vi "DTMF_final_rev2.vi"() -> ()   [LabVIEW 2018]
uses:
  <vilib>/Analysis/3filter.llb/Filter Passband Type.ctl
  <vilib>/Analysis/5stat.llb/RMS (DBL).vi
  <vilib>/express/express analysis/Spectral/Block/exnSpectralBlock spectral measurements power poly.vi
  <vilib>/express/express analysis/Spectral/Block/exnSpectralBlock spectral measurements power WFM.vi
  <vilib>/Analysis/3filter.llb/Butterworth Filter (DBL).vi
  <vilib>/express/express analysis/Spectral/XNode/ExpressSpectralMeasurementsBlockNode.xnode
  <vilib>/Analysis/NI_AALPro.lvlib
  <vilib>/Analysis/NI_AALBase.lvlib
panel:
  out "Peaks":cluster{"f0":dbl, "df":dbl, "magnitude":dbl[]}(graph)
  out "Dectected Phone Number!":i32[](array[numeric])
  out "Current Piece of Waveform Graph":dbl[](graph)
  out "appended array 2":dbl[](array[numeric])
  out "Total Signals":dynamicdata(graph) caption="Signals"
  out "max index(es) 2":i32
  out "max index(es)":i32
  out "appended array":dbl[](array[numeric])
  out "rms value":dbl format="%0.2f"
  in  "Emergency Exit":bool
  out "File Directory":path
  # "Tom's Dual Tone Multi Frequency"
  # "<- Total Dialed Phone #"
  # "Represents\ntotal signal ->"
  # "867-5309"
  # "OU SWAG"
  # "<-  Represents two peaks \n      if the phone number \n      is pressed"
  # "Represents how the \nwaveform looks in\nthe graph            ->"
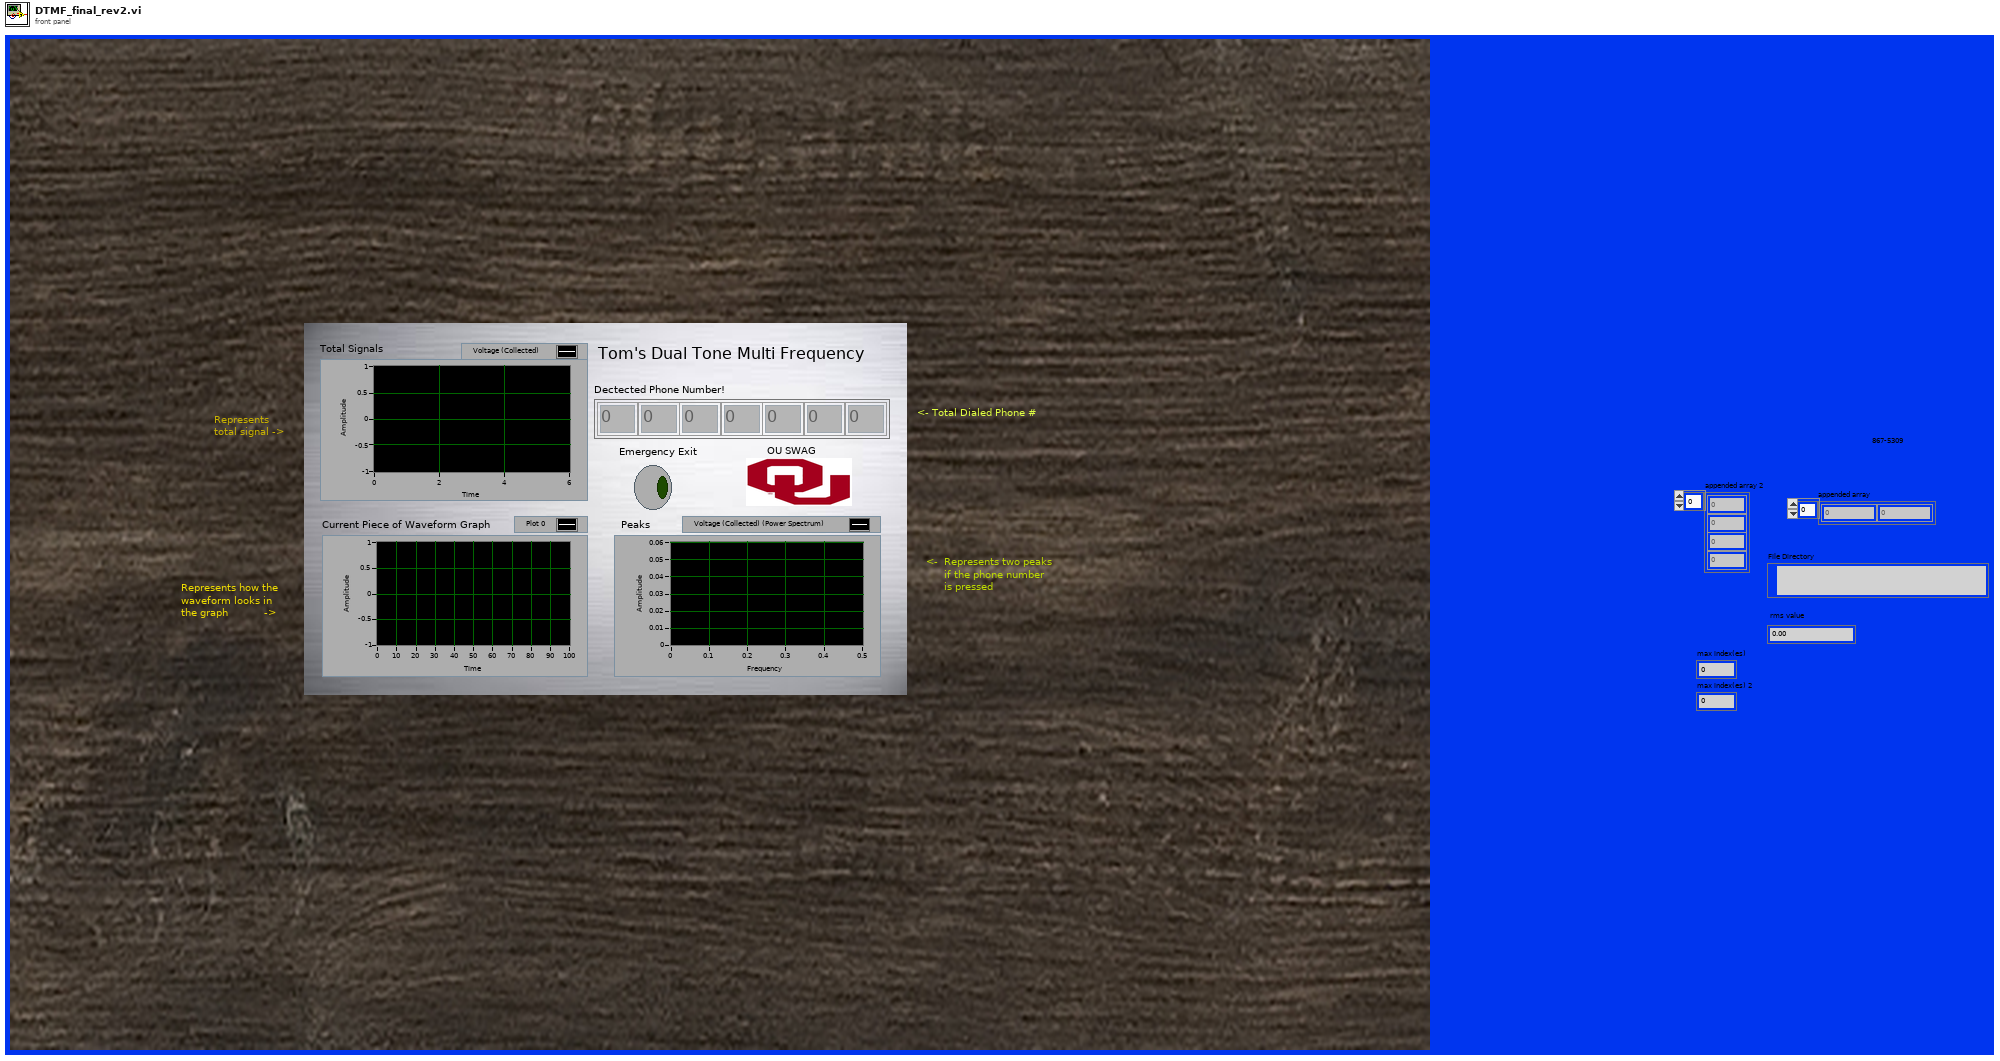
[diagram p1: front panel]
types:
  T1 = cluster{"averaging mode":u16, "weighting mode":u16, "number of averages":u32}
  T2 = cluster{"dB On (F)":bool, "unwrap phase (F)":bool, "convert to degree (F)":bool}
  T3 = typedef "NI_AALBase.lvlib/Filter Passband Type.ctl" = enum32{"Lowpass", "Highpass", "Bandpass", "Bandstop"}
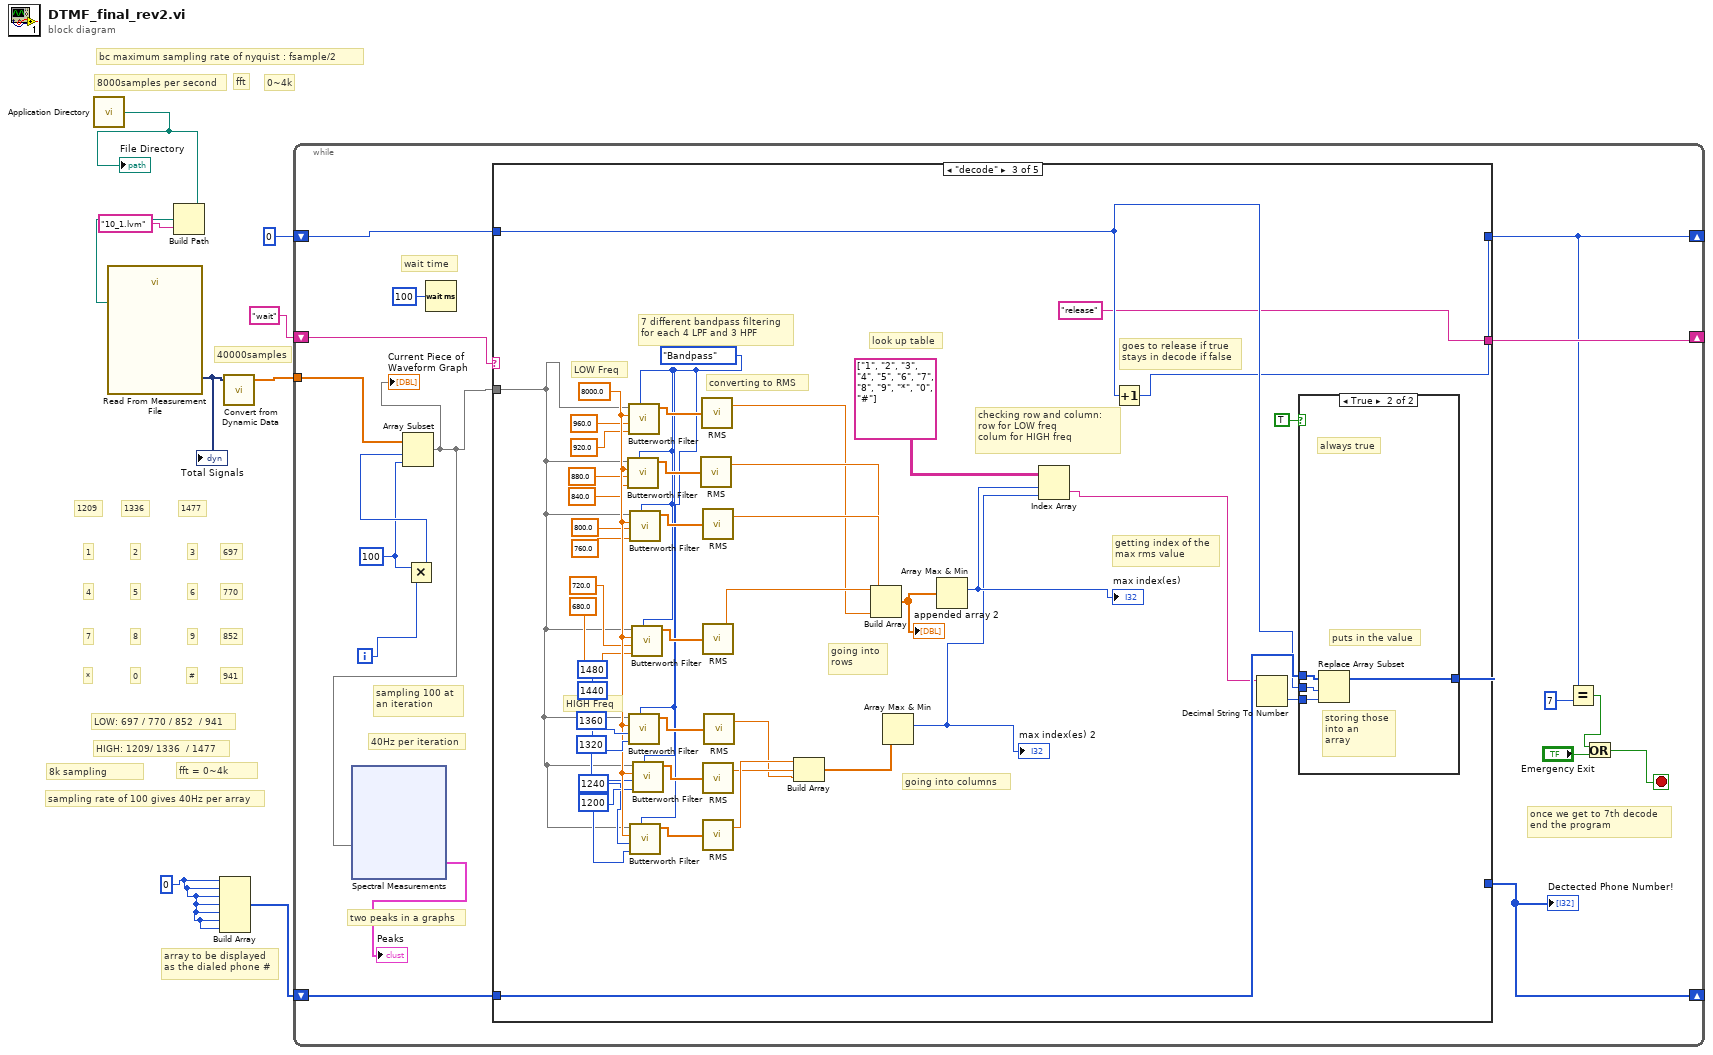
[diagram p0: block diagram]
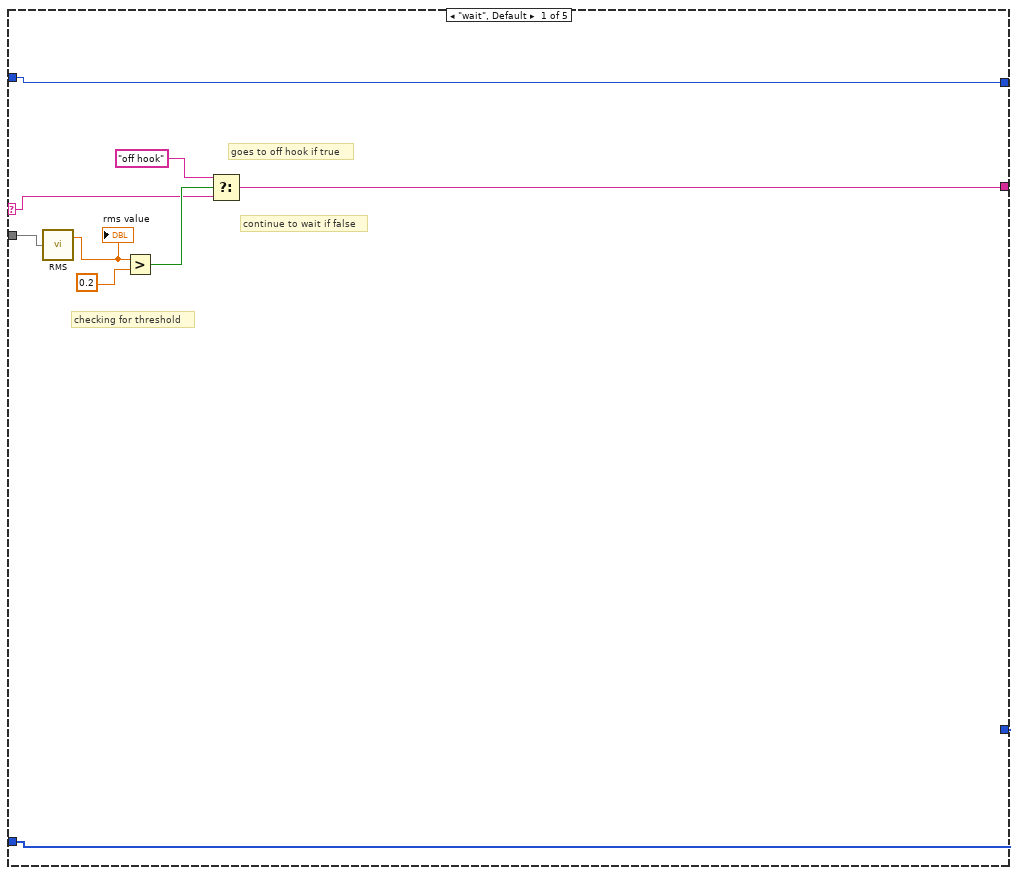
[diagram p2: hidden frame]
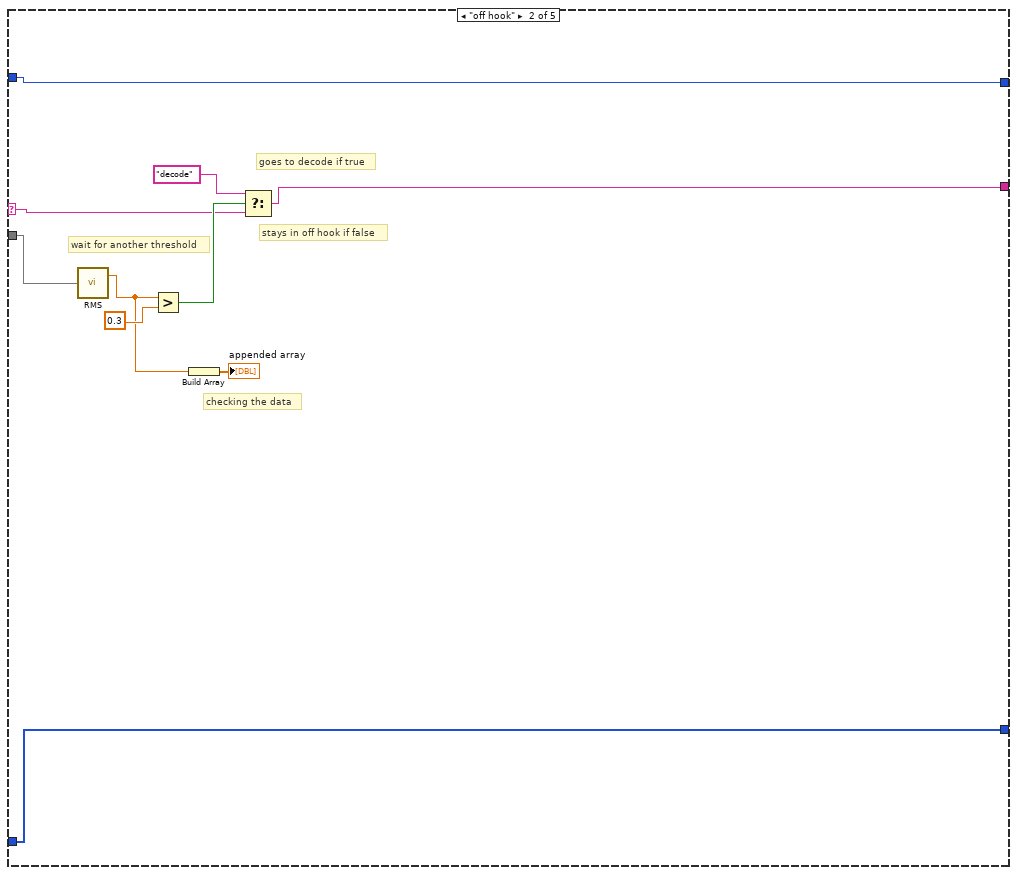
[diagram p3: hidden frame]
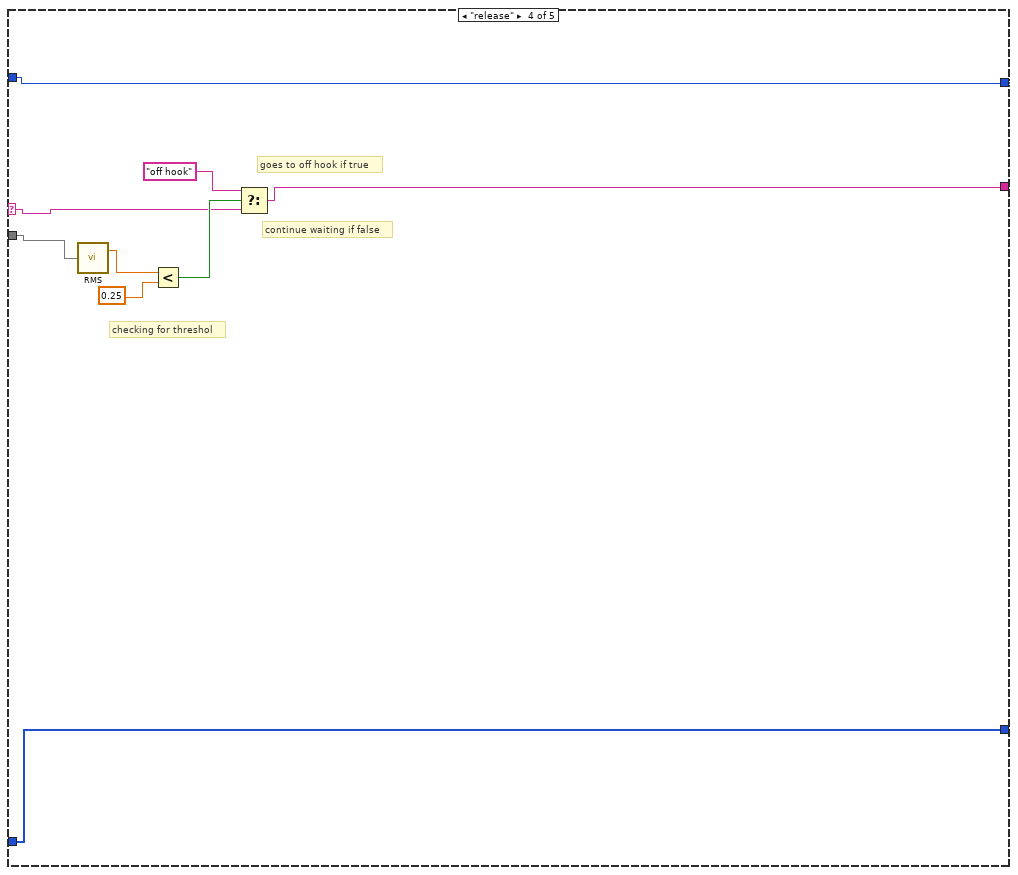
[diagram p5: hidden frame]
diagram:
  w1 = 0
  # "array to be displayed\nas the dialed phone #"
  # "sampling rate of 100 gives 40Hz per array"
  # "fft = 0~4k"
  # "8k sampling"
  # "HIGH: 1209/ 1336  / 1477"
  # "LOW: 697 / 770 / 852  / 941"
  # "40000samples"
  # "941"
  # "852"
  # "770"
  # "697"
  # "1477"
  # "1336"
  # "1209"
  # "#"
  # "0"
  # "*"
  # "9"
  # "8"
  # "7"
  # "6"
  # "5"
  # "4"
  # "3"
  # "2"
  # "1"
  # "bc maximum sampling rate of nyquist : fsample/2"
  # "0~4k"
  # "fft"
  # "8000samples per second"
  n1 = call <vilib>:"Application Directory.vi"() -> ("Application Directory"=w4:path)
  "File Directory" <- w4
  n2 = Build Path(base path=w4, name or relative path="10_1.lvm") -> (appended path=w3:path)
  n3 = call "Read From Measurement File"("Filename"=w3) -> ("Signals"=w9:dynamicdata)  [unwired: 5 in, 5 out]
  "Total Signals" <- w9
  n4 = Build Array(w1, w1, w1, w1, w1, w1, w1) -> (w2:i32[])
  n5 = call "Convert from Dynamic Data"("Dynamic Data Type"=w9) -> ("Array"=w8:dbl[])  [unwired: 3 in]
  n6 = while {
    tunnel: w8 -> [w24]
    shift-right: [w22] -> _
    shift-left: "wait" -> [w26]
    shift-right: [w17] -> _
    shift-left: 0 -> [w21]
    shift-right: [w10] -> _
    shift-left: w2 -> [w11]
    i -> [w25]
    stop <- w16 stop-if-true
    w12 = 100 ("x")
    # "wait time"
    # "two peaks in a graphs"
    # "40Hz per iteration"
    # "sampling 100 at \nan iteration"
    # "once we get to 7th decode\nend the program"
    n7 = Multiply(x=w12, y=w25) -> (x*y=w23:i32)
    n8 = Array Subset(array=w24, index=w23, length=w12) -> (w14:dbl[])
    "Current Piece of Waveform Graph" <- w14
    n9 = xnode "Spectral Measurements"("Signals"=w14) -> ("Power Spectrum"=→"Peaks":cluster{"f0":dbl, "df":dbl, "magnitude":dbl[]})  [unwired: 1 in, 1 out]
    n10 = Wait (ms)(milliseconds to wait=u32 100) -> ()  [unwired: 1 out]
    n11 = case shown="\"decode\"" w26 {
      selector: w26 -> [w40 w51 _ w108 w114]
      tunnel: w14 -> [w44 w50 w66 w107 _]
      tunnel: [w39 w49 "release" ("t") w106 w114] -> w22
      tunnel: w21 -> [w37 w48 w62 w105 w115]
      tunnel: [w37 w48 w57 w105 w115] -> w17
      tunnel: [w36 w45 w65 w104 w113] -> w10
      tunnel: w11 -> [w36 w45 w63 w104 w113]
      frame "wait", Default {
        # "checking for threshold"
        # "continue to wait if false"
        # "goes to off hook if true"
        n12 = call-poly <vilib>:"RMS.vi"("X"=w44) -> ("rms value"=w43:dbl)  [unwired: 1 out]
        "rms value" <- w43
        n13 = Greater?(x=w43, y=0.2) -> (0:w41:bool)
        n14 = Select(t="off hook", s=w41, f=w40) -> (s? t:f=w39:string)
      }
      frame "off hook" {
        # "stays in off hook if false"
        # "goes to decode if true"
        # "checking the data"
        # "wait for another threshold"
        n15 = call-poly <vilib>:"RMS.vi"("X"=w50) -> ("rms value"=w47:dbl)  [unwired: 1 out]
        n16 = Greater?(x=w47, y=0.3) -> (0:w53:bool)
        n17 = Build Array(w47) -> (→"appended array":dbl[])
        n18 = Select(t="decode", s=w53, f=w51) -> (s? t:f=w49:string)
      }
      frame "decode" {
        w74 = Filter_Passband_Type."Bandpass" ("filter type")
        w95 = 8000.0 ("sampling freq: fs")
        # "going into\nrows"
        # "going into columns"
        # "checking row and column:\nrow for LOW freq\ncolum for HIGH freq"
        # "look up table"
        # "goes to release if true\nstays in decode if false"
        # "HIGH Freq"
        # "LOW Freq"
        # "getting index of the\nmax rms value"
        # "converting to RMS"
        # "7 different bandpass filtering\nfor each 4 LPF and 3 HPF"
        n19 = call-poly <vilib>:"Butterworth Filter.vi"("filter type"=w74, "low cutoff freq: fl"=840.0 ("lower limit"), "high cutoff freq: fh"=880.0 ("lower limit"), "sampling freq: fs"=w95, "X"=w66) -> ("Filtered X"=w82:dbl[])  [unwired: 3 in, 1 out]
        n20 = call-poly <vilib>:"Butterworth Filter.vi"("filter type"=w74, "low cutoff freq: fl"=920.0 ("upper limit"), "high cutoff freq: fh"=960.0 ("lower limit"), "sampling freq: fs"=w95, "X"=w66) -> ("Filtered X"=w98:dbl[])  [unwired: 3 in, 1 out]
        n21 = call-poly <vilib>:"Butterworth Filter.vi"("filter type"=w74, "low cutoff freq: fl"=1440 ("lower limit"), "high cutoff freq: fh"=1480 ("lower limit"), "sampling freq: fs"=w95, "X"=w66) -> ("Filtered X"=w79:dbl[])  [unwired: 3 in, 1 out]
        n22 = call-poly <vilib>:"Butterworth Filter.vi"("filter type"=w74, "low cutoff freq: fl"=760.0 ("lower limit"), "high cutoff freq: fh"=800.0 ("lower limit"), "sampling freq: fs"=w95, "X"=w66) -> ("Filtered X"=w81:dbl[])  [unwired: 3 in, 1 out]
        n23 = call-poly <vilib>:"Butterworth Filter.vi"("filter type"=w74, "low cutoff freq: fl"=1200 ("lower limit"), "high cutoff freq: fh"=1240 ("lower limit"), "sampling freq: fs"=w95, "X"=w66) -> ("Filtered X"=w77:dbl[])  [unwired: 3 in, 1 out]
        n24 = call-poly <vilib>:"Butterworth Filter.vi"("filter type"=w74, "low cutoff freq: fl"=680.0 ("lower limit"), "high cutoff freq: fh"=720.0 ("lower limit"), "sampling freq: fs"=w95, "X"=w66) -> ("Filtered X"=w80:dbl[])  [unwired: 3 in, 1 out]
        n25 = call-poly <vilib>:"Butterworth Filter.vi"("filter type"=w74, "low cutoff freq: fl"=1320 ("lower limit"), "high cutoff freq: fh"=1360 ("lower limit"), "sampling freq: fs"=w95, "X"=w66) -> ("Filtered X"=w78:dbl[])  [unwired: 3 in, 1 out]
        n26 = call-poly <vilib>:"RMS.vi"("X"=w82) -> ("rms value"=w68:dbl)  [unwired: 1 out]
        n27 = call-poly <vilib>:"RMS.vi"("X"=w98) -> ("rms value"=w67:dbl)  [unwired: 1 out]
        n28 = call-poly <vilib>:"RMS.vi"("X"=w81) -> ("rms value"=w69:dbl)  [unwired: 1 out]
        n29 = call-poly <vilib>:"RMS.vi"("X"=w80) -> ("rms value"=w70:dbl)  [unwired: 1 out]
        n30 = call-poly <vilib>:"RMS.vi"("X"=w78) -> ("rms value"=w72:dbl)  [unwired: 1 out]
        n31 = call-poly <vilib>:"RMS.vi"("X"=w77) -> ("rms value"=w73:dbl)  [unwired: 1 out]
        n32 = call-poly <vilib>:"RMS.vi"("X"=w79) -> ("rms value"=w71:dbl)  [unwired: 1 out]
        n33 = Build Array(w73, w72, w71) -> (w75:dbl[])
        n34 = Build Array(w70, w69, w68, w67) -> (w76:dbl[])
        "appended array 2" <- w76
        n35 = Array Max & Min(array=w75) -> (max index (indices)=w60:i32)  [unwired: 3 out]
        "max index(es) 2" <- w60
        n36 = Array Max & Min(array=w76) -> (max index (indices)=w61:i32)  [unwired: 3 out]
        "max index(es)" <- w61
        n37 = Index Array(array=string[][] [["1", "2", "3"], ["4", "5", "6"], ["7", "8", "9"], ["*", "0", "#"]], index (row)=w61, index (col)=w60) -> (element=w59:string)
        n38 = Increment(x=w62) -> (x+1=w57:i32)
        n39 = Decimal String To Number(string=w59) -> (number=w64:i32)  [unwired: 2 in, 1 out]
        n40 = case shown="True" TRUE {
          tunnel: [w99 w103] -> w65
          tunnel: w64 -> [_ w101]
          tunnel: w63 -> [w99 w102]
          tunnel: w62 -> [_ w100]
          frame False {
          }
          frame True {
            # "storing those\ninto an\narray"
            # "puts in the value"
            # "always true"
            n41 = Replace Array Subset(array=w102, new element=w101, index=w100) -> (w103:i32[])
          }
        }
      }
      frame "release" {
        # "continue waiting if false"
        # "goes to off hook if true"
        # "checking for threshol"
        n42 = call-poly <vilib>:"RMS.vi"("X"=w107) -> ("rms value"=w112:dbl)  [unwired: 1 out]
        n43 = Less?(x=w112, y=0.25) -> (x < y?=w110:bool)
        n44 = Select(t="off hook", s=w110, f=w108) -> (s? t:f=w106:string)
      }
      frame "end" {
        # "going through~"
        # "going through~"
      }
    }
    "Dectected Phone Number!" <- w10
    n45 = Equal?(x=w17, y=7) -> (x = y?=w19:bool)
    n46 = Or(x=w19, y="Emergency Exit") -> (x .or. y?=w16:bool)
  }
